vi "Pelletron_Controller.vi"() -> ()   [LabVIEW 2013, in "AccelNET.lvlib" / "Control_VIs.lvlib"]
uses:
  Device IO/Pelletron/Accelnet/Control_VIs.lvlib
  Device IO/Pelletron/Accelnet/Component_Power_Indicator.ctl
  Device IO/Pelletron/Accelnet/Interlocks.ctl
  Device IO/Pelletron/Accelnet/Bypass_Indicator.ctl
  Device IO/Pelletron/Accelnet/Parameters_Indicator.ctl
  Device IO/Pelletron/Accelnet/Parameters_Control.ctl
  Device IO/Pelletron/Accelnet/Conditioning.ctl
  Device IO/Pelletron/Accelnet/Component_Power_Control.ctl
  Device IO/Pelletron/Accelnet/Bypass_Control.ctl
  Controls/PelletronLabview.ctl
  <vilib>/Utility/miscctls.llb/LVPointTypeDef.ctl
  Device IO/Pelletron/Accelnet/TCPinfo.vi
  <userlib>/_OpenG.lib/comparison/comparison.llb/Variant Changed__ogtk.vi
  Device IO/Pelletron/Accelnet/TCP.lvclass
  Device IO/Pelletron/Accelnet/Global_Variables.lvlib
  Device IO/Pelletron/Accelnet/Useful_SubVIs.lvlib
  Device IO/Pelletron/Accelnet/Useful_Controls.lvlib
panel:
  in  "Shut Down":bool
  out "uA/kV":dbl
  in  "Post to database?":bool=TRUE
  out "Connection Status":bool
  out "Bypass Turn Off":dbl format="%<%H:%M:%S>t"
  in  "Synch":bool
  out "Interlock Status":T1
  in  "Y Log Scale?":bool
  in  "X Maximum":dbl max=0.0 step=30.0 format="%<%H:%M:%S>t"
  in  "X Autoscale":bool=TRUE
  in  "X Minimum":dbl max=0.0 step=30.0 format="%<%H:%M:%S>t"
  in  "Y Autoscale":bool=TRUE
  in  "Y Maximum":dbl
  in  "Y Minimum":dbl
  out "Start Time":dbl format="%<%m/%d/%Y  -  %H:%M:%S>T"
  in  "Clear":bool
  out "XY Graph":cluster{dbl[], dbl[]}(graph)
  in  "Plotter Selector":u16(ring) items=["High Voltage", "High Voltage PS", "Chain Current", "Column Current", "Lost Charge", "Radiation", "Pressure", "HV Control Difference"]
  out "Stop Checking for Sparks Start":dbl
  in  "Stop Condition":bool
  in  "Spark Counter Reset":bool
  in  "Update Parameters":bool
  in  "Param Controls":T2 {"Control Reference\nVoltage (MV)" min=0.3 max=3.0 step=0.1; "High Voltage\nPS Setting (kV)" min=0.0 max=18.0 step=0.2; "Spark\nLimit" min=0.0 max=10.0 step=1.0}
  out "Parameters":T3 {"High\nVoltage (MV)" format="%#.4g"; "Control Reference\nVoltage (MV)" format="%#.4g"; "+ High Voltage\nPS (kV)" format="%#.4g"; "- High Voltage\nPS (kV)" format="%#.4g"; "HV Control\nDifference (kV)" format="%#.4g"; "High Voltage\nPS Setting (kV)" format="%#.4g"; "Chain\nCurrent (uA)" format="%#.4g"; "Column\nCurrent (uA)" format="%#.4g"; "Spark\nLimit" format="%#.0g"; "Spark\nCount" format="%#.0g"; "Lost Charge (uA)" scale=-10.0..10.0; "Spark\nThreshold (MV)" format="%#.4g"; "Radiation (mRad/hr)" step=3.978696e-316 scale=0.02..200.0 scale format="%#.4f"; "Vacuum (Torr)" scale=1e-09..0.001 scale format="%#_6e"}
  out "Warning!":bool
  in  "Reset":bool
  out "Rad. Avg.":dbl(slide) scale=0.02..200.0 scale format="%.0e"
  out "Stopped":bool
  out "Spark\nCounter":i64
  in  "Spark Limit":i64=2
  in  "Emergency Stop":bool
  out "Accelnet Write Errors":errorcluster
  in  "Clear Errors":bool
  out "Accelnet Read Errors":errorcluster
  in  "stop":bool
  out "Condition\nStart Time":dbl format="%<%H:%M:%S>T"
  in  "Conditioning":T4
  in  "Bypass Control":T5
  in  "Update Bypass":bool
  out "Pelletron Bypass":T6
  in  "Component Power Control":T7
  in  "Update On/off":bool
  out "Component\nPower":T8
  # "Instructions:\n\n1) Make sure TCP Control is on and the connection is open.  This is true if you can see TCP information on the top where it says IP Address.\n\n2) Turn on the Pelletron Controller\n\n3) Check to see that the Blower and Ion Gauge Filament is on\n\n4) Check all interlocks are lighte and all bypasses are not.\n\n5) Controls are separate from readings.  Pressing the update button in each respective section sends the commands to the Accelnet system.\n\n6) If the Stopped light is on, then the system will lock out all Pelletron controls and shut off the system until the Reset button is pressed.\n\n7) When finished, stop program with Stop button (make sure Pelletron is off)."
  # "Pelletron Startup Sequence:\n1.  Turn on HV Power Supply\n2. Check +High Voltage PS under parameters to be 1 kV if not change it using the High Voltage PS Setting\n3. Turn on Chain PS\n4. Turn on Chain\n5. Condition Pelletron using auto conditioner or manually using High Voltage PS Setting under Parameter Control\n6.  Check Control Reference Voltage under Parameters to be desired voltage and change it if it is not\n7.  Turn on Control Mode\n8.  Open Beamline Gate Valve\n9.  Turn on Rotating Shaft\n10. Operate Pelletron source through Andrew's Box"
  # "Pelletron Shutdown Sequence:\n1.  Make sure Andrew's box is turned down and off\n2.  Turn off Rotating Shaft\n3.  Close Beamline Gatevalve\n         a.  If you are leaving the pelletron on but the accelerator off, stop here.\n4. Check High Voltage PS Setting to be close to + High Voltage PS, if not set it to ~0.2kV above the current setting\n5.  Turn off Control Mode\n6.  Set Voltage to 1 kv using HighVoltage PS Setting\n7.  Reset spark counter after you see the spark count rise by one by hitting the Spark Reset Button.\n8.  Turn off Chain\n9.  Turn off Chain PS and HV Power Supply\n10.  Stop the program."
  # "Interlocks"
  # "Pelletron Plotter"
  # "Parameter Control"
  # "Parameters"
  # "LabVIEW Interlocks"
  # "Pelletron\n   Stop"
  # "Conditioning"
  # "Bypass"
  # "Component On/Off"
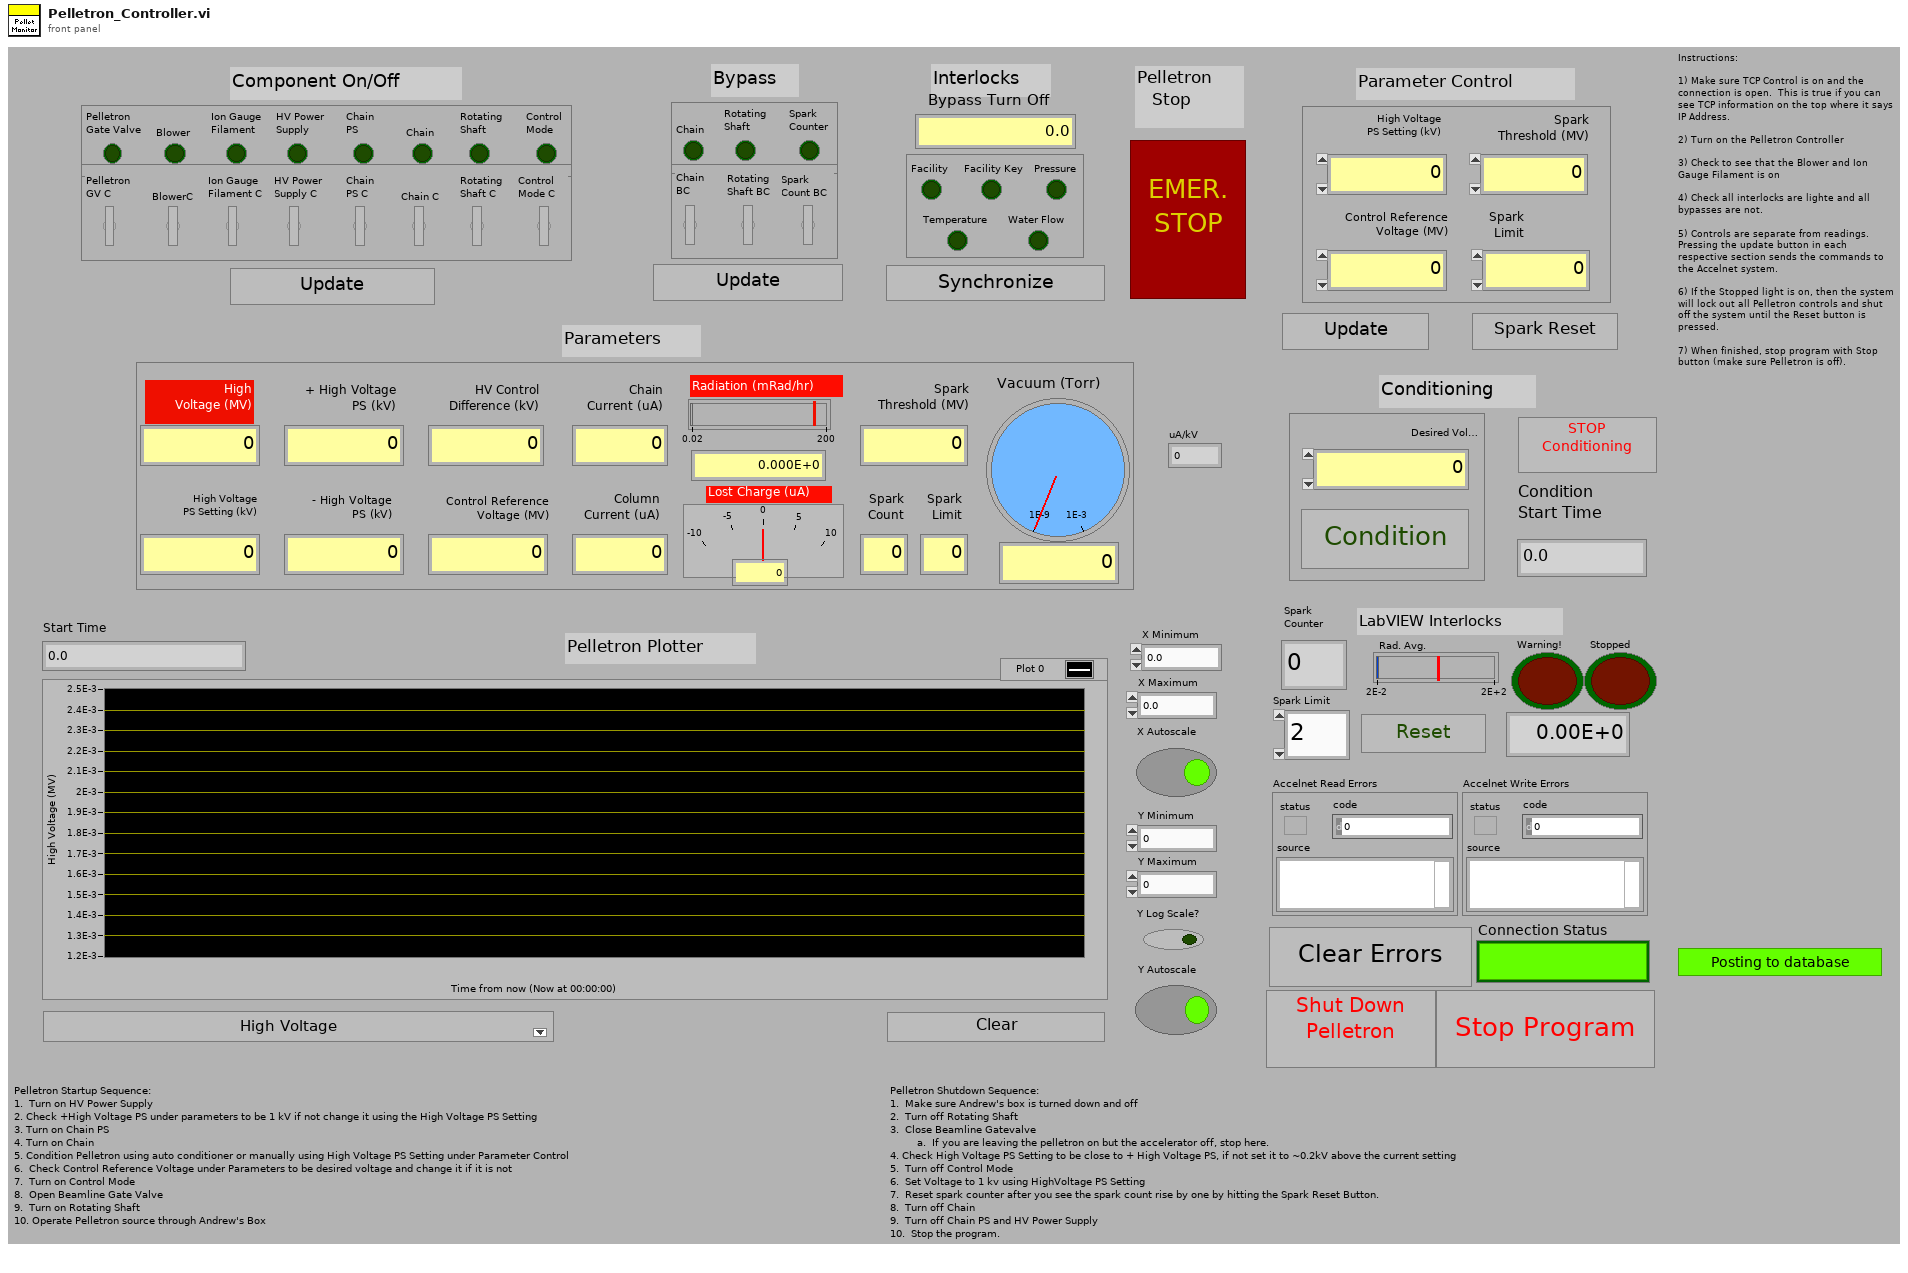
[diagram p1: front panel]
types:
  T1 = typedef "AccelNET.lvlib/Useful_Controls.lvlib/Interlocks.ctl" = cluster{"Facility":bool, "Facility Key":bool, "Water Flow":bool, "Pressure":bool, "Temperature":bool}
  T2 = typedef "AccelNET.lvlib/Useful_Controls.lvlib/Parameters_Control.ctl" = cluster{"Spark\nThreshold (MV)":dbl, "Spark\nLimit":dbl, "High Voltage\nPS Setting (kV)":dbl, "Control Reference\nVoltage (MV)":dbl}
  T3 = typedef "AccelNET.lvlib/Useful_Controls.lvlib/Parameters_Indicator.ctl" = cluster{"Vacuum (Torr)":dbl, "Radiation (mRad/hr)":dbl, "Spark\nThreshold (MV)":dbl, "Lost Charge (uA)":dbl, "Spark\nCount":dbl, "Spark\nLimit":dbl, "Column\nCurrent (uA)":dbl, "Chain\nCurrent (uA)":dbl, "High Voltage\nPS Setting (kV)":dbl, "HV Control\nDifference (kV)":dbl, "- High Voltage\nPS (kV)":dbl, "+ High Voltage\nPS (kV)":dbl, "Control Reference\nVoltage (MV)":dbl, "High\nVoltage (MV)":dbl}
  T4 = typedef "AccelNET.lvlib/Useful_Controls.lvlib/Conditioning.ctl" = cluster{"Desired Voltage (MV)":dbl, "Conditioning?":bool}
  T5 = typedef "AccelNET.lvlib/Useful_Controls.lvlib/Bypass_Control.ctl" = cluster{"Chain\nBC":bool, "Rotating\nShaft BC":bool, "Spark\nCount BC":bool}
  T6 = typedef "AccelNET.lvlib/Useful_Controls.lvlib/Bypass_Indicator.ctl" = cluster{"Chain":bool, "Rotating\nShaft":bool, "Spark\nCounter":bool}
  T7 = typedef "AccelNET.lvlib/Useful_Controls.lvlib/Component_Power_Control.ctl" = cluster{"Pelletron\nGV C":bool, "BlowerC":bool, "Chain C":bool, "Rotating\nShaft C":bool, "HV Power\nSupply C":bool, "Ion Gauge\nFilament C":bool, "Control\nMode C":bool, "Chain\nPS C":bool}
  T8 = typedef "AccelNET.lvlib/Useful_Controls.lvlib/Component_Power_Indicator.ctl" = cluster{"Pelletron\nGate Valve":bool, "Blower":bool, "Chain":bool, "Rotating\nShaft":bool, "HV Power\nSupply":bool, "Ion Gauge\nFilament":bool, "Control\nMode":bool, "Chain\nPS":bool}
  T9 = typedef "LVPointTypeDef.ctl" = cluster{"Horizontal":i16, "Vertical":i16}
  T10 = typedef "PelletronLabview.ctl" = cluster{"Timestamp":timestamp, "High Voltage":sgl, "+ High Voltage Supply":dbl, "- High Voltage Supply":dbl, "HV Control Difference":dbl, "Vacuum Pressure":sgl, "Radiation":dbl, "Column Current":sgl, "Lost Charge":dbl, "Chain Current":sgl, "Control High Voltage":dbl}
  T11 = cluster{"Time":dbl, "High Voltage":dbl, "High VoltagePS":dbl, "Chain Current":dbl, "Column Current":dbl, "Lost Charge":dbl, "Radiation":dbl, "Pressure":dbl, "HV Control Difference":dbl}[]
  T12 = cluster{"Spark\nThreshold (MV)":dbl, "Spark\nLimit":dbl, "High Voltage\nPS Setting (kV)":dbl, "Control Reference\nVoltage (MV)":dbl}
  T13 = enum8{"Enabled", "Disabled", "Disabled and Grayed Out"}
  T14 = cluster{"Time":dbl, "High Voltage":dbl, "High VoltagePS":dbl, "Chain Current":dbl, "Column Current":dbl, "Lost Charge":dbl, "Radiation":dbl, "Pressure":dbl, "HV Control Difference":dbl}
  T15 = cluster{"High\nVoltage (MV)":dbl, "Vacuum (Torr)":dbl, "Lost Charge (uA)":dbl, "+ High Voltage\nPS (kV)":dbl}
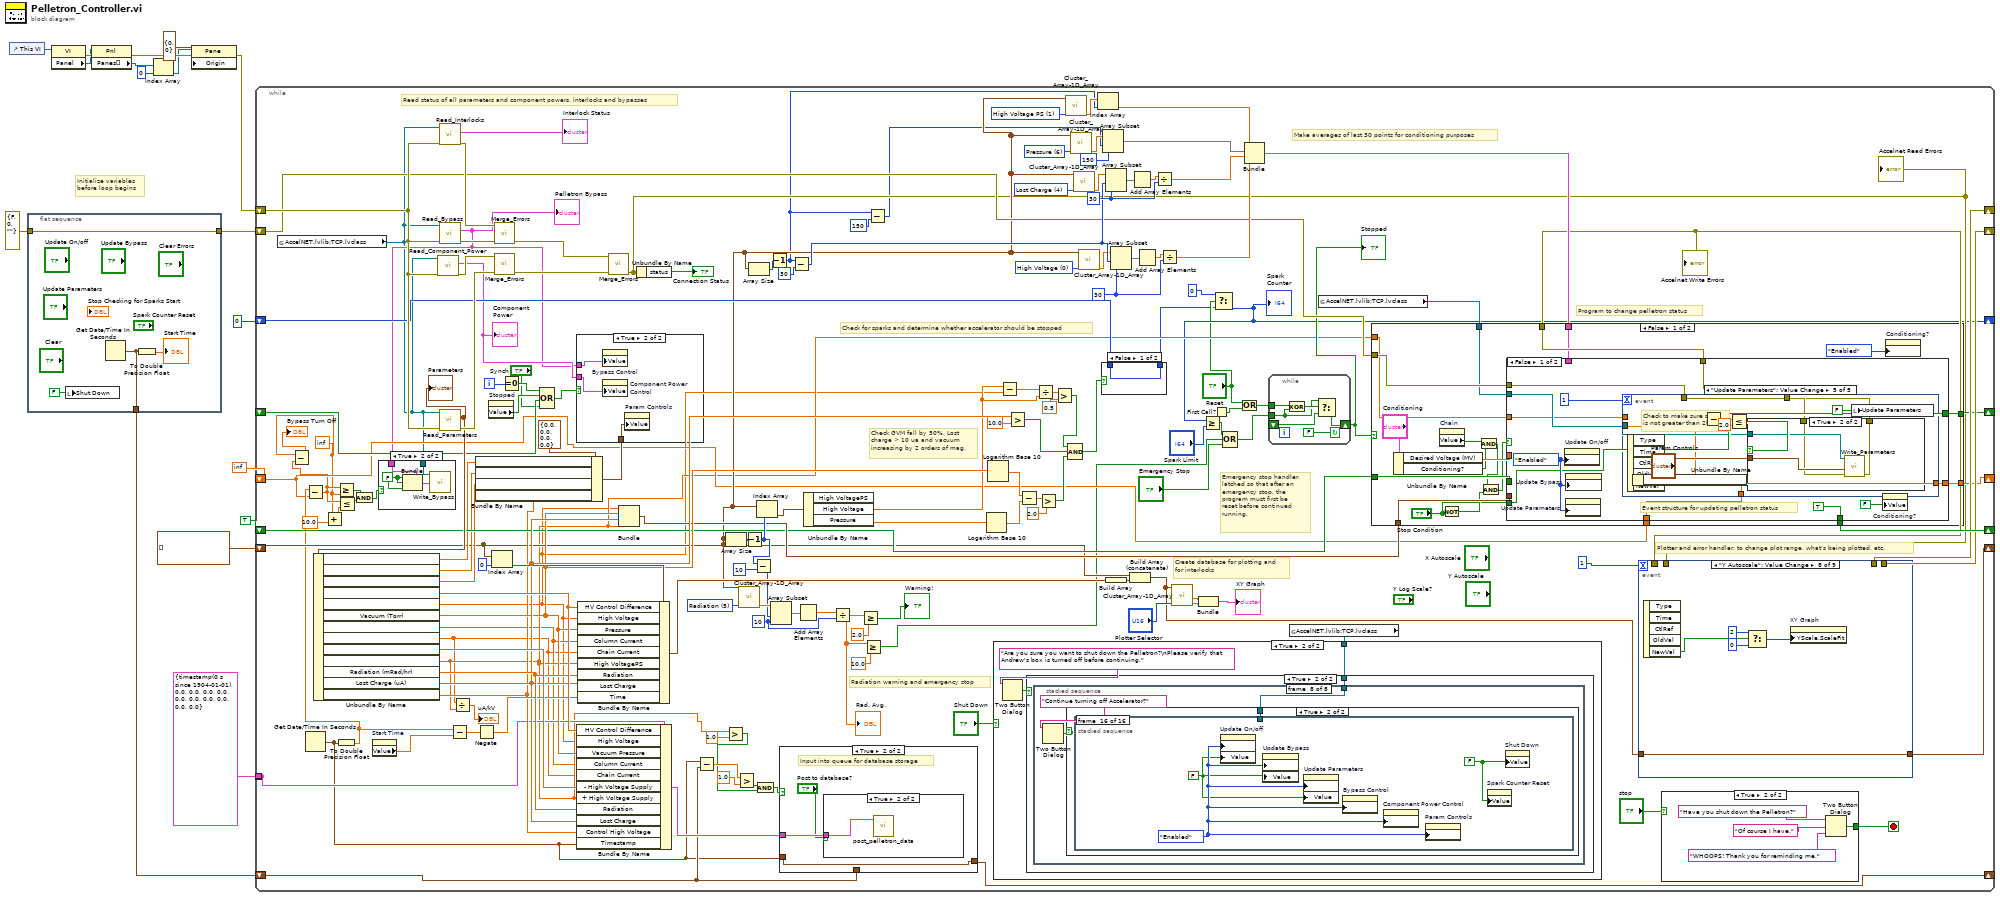
[diagram p0: block diagram]
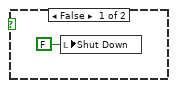
[diagram p3: hidden frame]
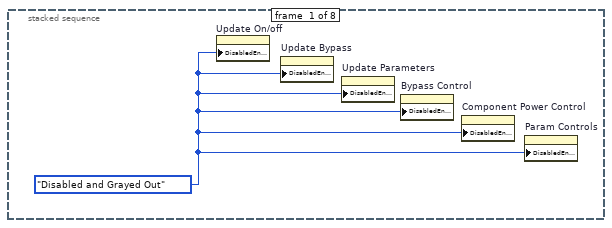
[diagram p4: hidden frame]
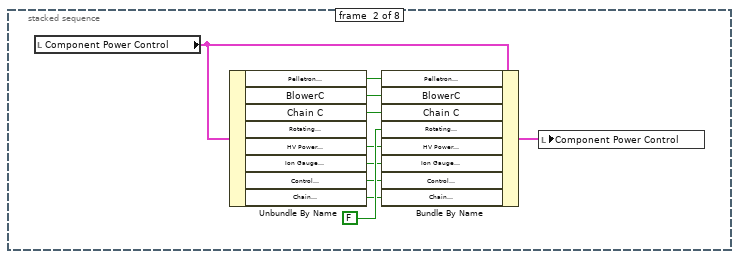
[diagram p5: hidden frame]
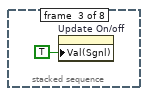
[diagram p6: hidden frame]
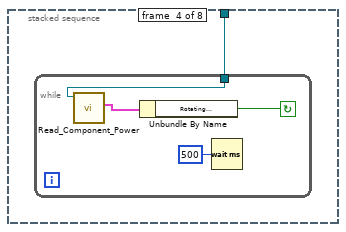
[diagram p7: hidden frame]
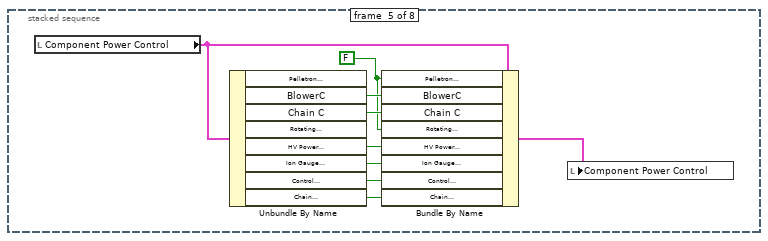
[diagram p8: hidden frame]
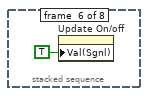
[diagram p9: hidden frame]
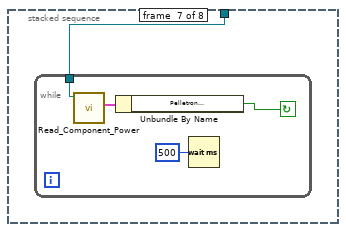
[diagram p10: hidden frame]
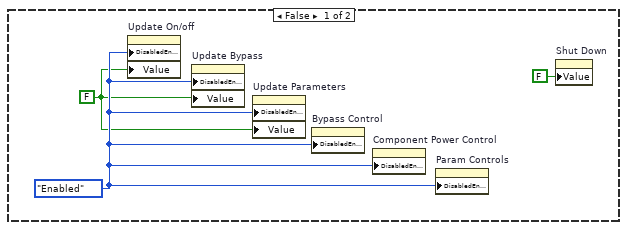
[diagram p11: hidden frame]
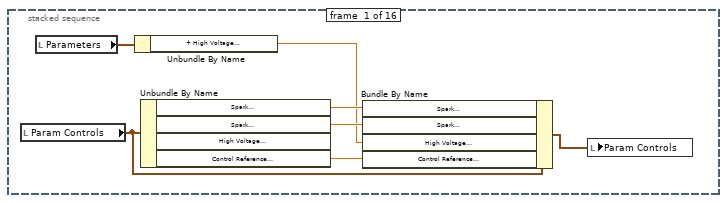
[diagram p12: hidden frame]
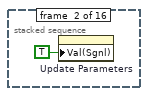
[diagram p13: hidden frame]
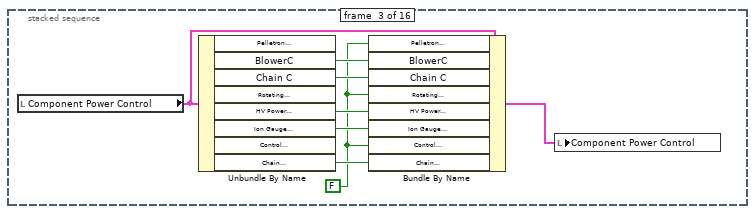
[diagram p14: hidden frame]
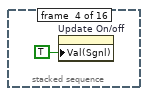
[diagram p15: hidden frame]
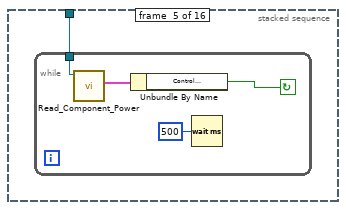
[diagram p16: hidden frame]
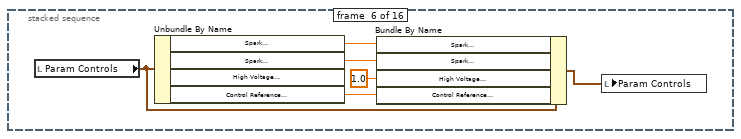
[diagram p17: hidden frame]
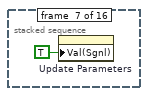
[diagram p18: hidden frame]
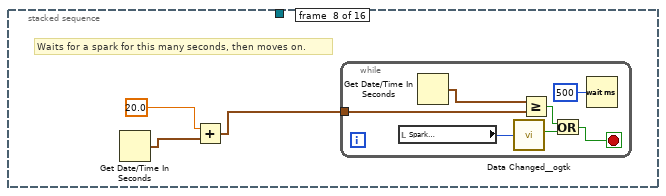
[diagram p19: hidden frame]
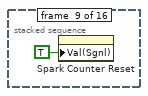
[diagram p20: hidden frame]
diagram:
  # "Initialize variables\nbefore loop begins"
  n1 = control-ref of="This VI"() -> (w12:refnum<vi>)
  n2 = flat-sequence {
    tunnel: [w21] -> w1
    tunnel: [w19] -> w2
    tunnel: errorcluster {"status"=FALSE, "code"=0, "source"=""} ("error out") -> [w21]
    frame #0 {
      n3 = local write "Shut Down"(FALSE ("Shut Down")) -> ()
      n4 = Get Date/Time In Seconds() -> (seconds since 1Jan1904=w19:timestamp)
      n5 = To Double Precision Float(number=w19) -> (double precision float=→"Start Time":dbl)
    }
  }
  n6 = property class="VI"(reference=w12) -> (error out=w11:errorcluster, "Panel"=w10:refnum<vi>)  [unwired: 1 in, 1 out]
  n7 = property class="Pnl"(reference=w10, error in=w11) -> (error out=w9:errorcluster, "Panes[]"=w8:refnum<vi>[])  [unwired: 1 out]
  n8 = Index Array(array=w8, index=0) -> (element=w6:refnum<vi>)
  n9 = property class="Pane"(reference=w6, error in=w9, "Origin"=T9 {"Horizontal"=0, "Vertical"=0}) -> (error out=w4:errorcluster)  [unwired: 1 out]
  n10 = while {
    shift-right: [w108] -> _
    shift-left: w4 -> [w174]
    shift-right: [w159] -> _
    shift-left: T11 [] -> [w92]
    shift-right: [w26] -> _
    shift-left: i64 0 -> [w138]
    shift-right: [w107] -> _
    shift-left: w1 -> [w97]
    shift-right: [w111] -> _
    shift-left: TRUE -> [w112]
    shift-right: [w70] -> _
    shift-left: _ -> [w69]
    shift-right: [w67] -> _
    shift-left: inf -> [w65]
    tunnel: [w48] -> _
    tunnel: T10 {"Timestamp"=timestamp(0 s since 1904-01-01), "High Voltage"=0.0, "+ High Voltage Supply"=0.0, "- High Voltage Supply"=0.0, "HV Control Difference"=0.0, "Vacuum Pressure"=0.0, "Radiation"=0.0, "Column Current"=0.0, "Lost Charge"=0.0, "Chain Current"=0.0, "Control High Voltage"=0.0} ("Cluster") -> [w48]
    shift-right: [w30] -> _
    shift-left: w2 -> [w44]
    i -> [w106]
    stop <- w29 stop-if-true
    w52 = inf ("y")
    w114 = u16 1 items=["High Voltage", "High Voltage PS", "Chain Current", "Column Current", "Lost Charge", "Radiation", "Pressure", "HV Control Difference"] ("Plotter Selector")
    w123 = u16 6 items=["High Voltage", "High Voltage PS", "Chain Current", "Column Current", "Lost Charge", "Radiation", "Pressure", "HV Control Difference"] ("Plotter Selector")
    w124 = 30 ("length")
    w127 = u16 4 items=["High Voltage", "High Voltage PS", "Chain Current", "Column Current", "Lost Charge", "Radiation", "Pressure", "HV Control Difference"] ("Plotter Selector")
    w130 = 30 ("length")
    w135 = u16 0 items=["High Voltage", "High Voltage PS", "Chain Current", "Column Current", "Lost Charge", "Radiation", "Pressure", "HV Control Difference"] ("Plotter Selector")
    w134 = 10 ("length")
    w148 = u16 5 items=["High Voltage", "High Voltage PS", "Chain Current", "Column Current", "Lost Charge", "Radiation", "Pressure", "HV Control Difference"] ("Plotter Selector")
    # "Emergency stop handler,\nlatched so that after an\nemergency stop, the \nprogram must first be \nreset before continued\nrunning."
    # "Plotter and error handler, to change plot range, what's being plotted, etc."
    # "Program to change pelletron status"
    # "Make averages of last 30 points for conditioning purposes"
    # "Check GVM fall by 50%, Lost\ncharge > 10 ua and vacuum\nincreasing by 2 orders of mag."
    # "Create database for plotting and\nfor interlocks"
    # "Radiation warning and emergency stop"
    # "Check for sparks and determine whether accelerator should be stopped"
    # "Read status of all parameters and component powers, interlocks and bypasses"
    n11 = global read "TCPinfo.vi" "AccelNET.lvlib:TCP.lvclass"() -> (w61:refnum<class "TCP.lvclass">)
    n12 = Get Date/Time In Seconds() -> (seconds since 1Jan1904=w43:timestamp)
    n13 = Add(x=w52, y=10.0) -> (x+y=w54:dbl)
    n14 = To Double Precision Float(number=w43) -> (double precision float=w66:dbl)
    n15 = Subtract(x=w66, y=w65) -> (x-y=w59:dbl)
    n16 = Subtract(x=w52, y=w59) -> (x-y=→"Bypass Turn Off":dbl)
    n17 = Greater Or Equal?(x=w59, y=w52) -> (x >= y?=w64:bool)
    n18 = Less Or Equal?(x=w59, y=w54) -> (x <= y?=w63:bool)
    n19 = And(x=w64, y=w63) -> (x .and. y?=w55:bool)
    n20 = property on="Start Time" class="DigNum (strict)"() -> ("Value"=w167:dbl)  [unwired: 2 in, 2 out]
    n21 = call "Read_Component_Power.vi"("error in (no error)"=w174, "AccelNET.lvlib:TCP.lvclass"=w61) -> ("Error Out"=w171:errorcluster, "Component Power"=w68:T8)  [unwired: 8 in]
    "Component\nPower" <- w68
    n22 = call "Read_Interlocks.vi"("Error In"=w174, "AccelNET.lvlib:TCP.lvclass"=w61) -> ("Error Out"=w173:errorcluster, "Interlock Status"=→"Interlock Status":T1)  [unwired: 8 in]
    n23 = call "Read_Bypass.vi"("error in (no error)"=w174, "AccelNET.lvlib:TCP.lvclass"=w61) -> ("Error Out"=w172:errorcluster, "Pelletron Bypass"=w62:T6)  [unwired: 8 in]
    "Pelletron Bypass" <- w62
    n24 = case shown="True" w55 {
      tunnel: w62 -> [_ w301]
      tunnel: w61 -> [_ w298]
      frame False {
      }
      frame True {
        w300 = FALSE ("Chain")
        n25 = Bundle(cluster=w301, "Chain"=w300, "Rotating\nShaft"=w300, "Spark\nCounter"=w300) -> (w299:T6)
        n26 = call "Write_Bypass.vi"("AccelNET.lvlib:TCP.lvclass"=w298, "Pelletron Bypass"=w299) -> ()  [unwired: 8 in, 1 out]
      }
    }
    n27 = call "Read_Parameters.vi"("error in (no error)"=w174, "AccelNET.lvlib:TCP.lvclass"=w61) -> ("Error Out"=w170:errorcluster, "Parameters"=w165:T3)  [unwired: 8 in]
    "Parameters" <- w165
    n28 = Unbundle By Name(w165) -> ("Spark\nThreshold (MV)"=w99:dbl, "Spark\nLimit"=w100:dbl, "High Voltage\nPS Setting (kV)"=w101:dbl, "HV Control\nDifference (kV)"=w153:dbl, "High\nVoltage (MV)"=w34:dbl, "Vacuum (Torr)"=w116:dbl, "Column\nCurrent (uA)"=w36:dbl, "Chain\nCurrent (uA)"=w35:dbl, "- High Voltage\nPS (kV)"=w154:dbl, "+ High Voltage\nPS (kV)"=w38:dbl, "Radiation (mRad/hr)"=w152:dbl, "Lost Charge (uA)"=w117:dbl, "Control Reference\nVoltage (MV)"=w102:dbl)
    n29 = Subtract(x=w66, y=w167) -> (x-y=w156:dbl)
    n30 = Divide(x=w35, y=w38) -> (x/y=→"uA/kV":dbl)
    n31 = Bundle By Name(cluster=T12 {"Spark\nThreshold (MV)"=0.0, "Spark\nLimit"=0.0, "High Voltage\nPS Setting (kV)"=0.0, "Control Reference\nVoltage (MV)"=0.0}, "Spark\nThreshold (MV)"=w99, "Spark\nLimit"=w100, "High Voltage\nPS Setting (kV)"=w101, "Control Reference\nVoltage (MV)"=w102) -> (w103:T12)
    n32 = Negate(x=w156) -> (-x=w151:dbl)
    n33 = property on="Stopped" class="Bool (strict)"() -> ("Value"=w77:bool)  [unwired: 2 in, 2 out]
    n34 = Index Array(array=w92, index=0) -> (element=w157:T14)
    n35 = call "Merge_Errors.vi"("Error 2"=w172, "Error 1"=w173) -> ("Error Out"=w169:errorcluster)  [unwired: 9 in]
    n36 = call "Merge_Errors.vi"("Error 2"=w170, "Error 1"=w171) -> ("Error Out"=w168:errorcluster)  [unwired: 9 in]
    n37 = Equal To 0?(x=w106) -> (x = 0?=w76:bool)
    n38 = Compound Arithmetic op=OR(w76, w77, w69, "Synch") -> (w75:bool)
    n39 = case shown="True" w75 {
      tunnel: w68 -> [_ w309]
      tunnel: w62 -> [_ w310]
      tunnel: w103 -> [_ w308]
      frame False {
      }
      frame True {
        n40 = property on="Bypass Control" class="Clust (strict)"("Value"=w310) -> ()  [unwired: 2 in, 2 out]
        n41 = property on="Component Power Control" class="Clust (strict)"("Value"=w309) -> ()  [unwired: 2 in, 2 out]
        n42 = property on="Param Controls" class="Clust (strict)"("Value"=w308) -> ()  [unwired: 2 in, 2 out]
      }
    }
    n43 = Bundle By Name(cluster=w48, "HV Control Difference"=w153, "High Voltage"=w34, "Vacuum Pressure"=w116, "Column Current"=w36, "Chain Current"=w35, "- High Voltage Supply"=w154, "+ High Voltage Supply"=w38, "Radiation"=w152, "Lost Charge"=w117, "Control High Voltage"=w102, "Timestamp"=w43) -> (w47:T10)
    n44 = Bundle By Name(cluster=w157, "HV Control Difference"=w153, "High Voltage"=w34, "Pressure"=w116, "Column Current"=w36, "Chain Current"=w35, "High VoltagePS"=w38, "Radiation"=w152, "Lost Charge"=w117, "Time"=w151) -> (w160:T14)
    n45 = call "Merge_Errors.vi"("Error 2"=w168, "Error 1"=w169) -> ("Error Out"=w57:errorcluster)  [unwired: 9 in]
    "Accelnet Read Errors" <- w57
    n46 = Bundle("High\nVoltage (MV)"=w34, "Vacuum (Torr)"=w116, "Lost Charge (uA)"=w117, "+ High Voltage\nPS (kV)"=w38) -> (w115:T15)  [unwired: 1 in]
    n47 = Unbundle By Name(w57) -> ("status"=→"Connection Status":bool)
    n48 = Subtract(x=w43, y=w44) -> (x-y=w45:dbl)
    n49 = Greater?(x=w38, y=1.0) -> (0:w40:bool)
    n50 = Array Size(array=w92) -> (size(s)=w150:i32)
    n51 = Greater?(x=w45, y=1.0 ("x")) -> (0:w42:bool)
    n52 = call "Cluster_Array-1D_Array.vi"("Plotter Selector"=w148, "Input Cluster"=w92) -> ("Output Data"=w147:dbl[])  [unwired: 8 in, 1 out]
    n53 = Decrement(x=w150) -> (x-1=w146:i32)
    n54 = Array Size(array=w92) -> (size(s)=w129:i32)
    n55 = Subtract(x=w146, y=10) -> (x-y=w133:i32)
    n56 = And(x=w42, y=w40) -> (x .and. y?=w41:bool)
    n57 = Index Array(array=w92, index=w146) -> (element=w149:T14)
    n58 = Decrement(x=w129) -> (x-1=w50:i32)
    n59 = Array Subset(array=w147, index=w133, length=w134) -> (w144:dbl[])
    n60 = case shown="True" w41 {
      tunnel: w47 -> [_ w296]
      tunnel: w44 -> [w293 _]
      tunnel: [w293 w295] -> w30
      tunnel: w43 -> [_ w295]
      frame False {
      }
      frame True {
        # "Input into queue for database storage"
        n61 = case shown="True" "Post to database?" {
          tunnel: w296 -> [_ w297]
          frame False {
          }
          frame True {
            n62 = call "post_pelletron_data.vi"("Input data"=w297) -> ()  [unwired: 9 in, 1 out]
          }
        }
      }
    }
    n63 = Subtract(x=w50, y=30) -> (x-y=w121:i32)
    n64 = Add Array Elements(numeric array=w144) -> (sum=w143:dbl)
    n65 = Unbundle By Name(w149) -> ("High Voltage"=w79:dbl, "Pressure"=w140:dbl)  [unwired: 1 out]
    n66 = Divide(x=w143, y=w134) -> (x/y=w98:dbl)
    "Rad. Avg." <- w98
    n67 = Greater Or Equal?(x=w98, y=2.0) -> (x >= y?=→"Warning!":bool)
    n68 = Greater Or Equal?(x=w98, y=10.0) -> (x >= y?=w32:bool)
    n69 = Subtract(x=w50, y=150) -> (x-y=w49:i32)
    n70 = Logarithm Base 10(1:w140) -> (0:w86:dbl)
    n71 = Logarithm Base 10(1:w116) -> (0:w87:dbl)
    n72 = Subtract(x=w79, y=w34) -> (x-y=w80:dbl)
    n73 = Greater?(x=w117, y=10.0) -> (0:w82:bool)
    n74 = Subtract(x=w87, y=w86) -> (x-y=w85:dbl)
    n75 = Divide(x=w80, y=w79) -> (x/y=w90:dbl)
    n76 = Greater?(x=w85, y=2.0) -> (0:w83:bool)
    n77 = Greater?(x=w90, y=0.5) -> (0:w81:bool)
    n78 = call "Cluster_Array-1D_Array.vi"("Plotter Selector"=w114, "Input Cluster"=w92) -> ("Output Data"=w71:dbl[])  [unwired: 8 in, 1 out]
    n79 = Compound Arithmetic op=AND(w81, w82, w83) -> (w139:bool)
    n80 = call "Cluster_Array-1D_Array.vi"("Plotter Selector"=w123, "Input Cluster"=w92) -> ("Output Data"=w72:dbl[])  [unwired: 8 in, 1 out]
    n81 = call "Cluster_Array-1D_Array.vi"("Plotter Selector"=w127, "Input Cluster"=w92) -> ("Output Data"=w73:dbl[])  [unwired: 8 in, 1 out]
    n82 = call "Cluster_Array-1D_Array.vi"("Plotter Selector"=w135, "Input Cluster"=w92) -> ("Output Data"=w74:dbl[])  [unwired: 8 in, 1 out]
    n83 = Index Array(array=w71, index=w50) -> (element=w113:dbl)
    n84 = case shown="False" w139 {
      tunnel: w138 -> [w431 w433]
      tunnel: [w431 w432] -> w24
      frame False {
      }
      frame True {
        n85 = Increment(x=w433) -> (x+1=w432:i64)
      }
    }
    n86 = Array Subset(array=w72, index=w49, length=150) -> (w91:dbl[])
    n87 = Array Subset(array=w73, index=w121, length=w124) -> (w126:dbl[])
    n88 = Build Array(w160) -> (w155:T11)
    n89 = Array Subset(array=w74, index=w121, length=w130) -> (w132:dbl[])
    n90 = Build Array (concatenate)(w92, w155) -> (w28:T11)
    n91 = Add Array Elements(numeric array=w126) -> (sum=w125:dbl)
    n92 = Add Array Elements(numeric array=w132) -> (sum=w131:dbl)
    n93 = Divide(x=w125, y=w124) -> (x/y=w120:dbl)
    n94 = Divide(x=w131, y=w130) -> (x/y=w119:dbl)
    n95 = call "Cluster_Array-1D_Array.vi"("Plotter Selector"="Plotter Selector", "Input Cluster"=w28) -> ("Output Data"=w163:dbl[], "Time"=w161:dbl[])  [unwired: 8 in]
    n96 = Bundle("Time"=w161, "Output Data"=w163) -> (→"XY Graph":cluster{"Time":dbl[], "Output Data":dbl[]})  [unwired: 1 in]
    n97 = First Call?() -> (First Call?: T/F=w94:bool)
    n98 = Select(t=i64 0, s="Reset", f=w24) -> (s? t:f=w26:i64)
    "Spark\nCounter" <- w26
    n99 = Greater Or Equal?(x=w26, y="Spark Limit") -> (x >= y?=w110:bool)
    n100 = Compound Arithmetic op=OR(w110, w32, "Emergency Stop") -> (w96:bool)
    n101 = Or(x="Reset", y=w94) -> (x .or. y?=w93:bool)
    n102 = Bundle("Vacuum (Torr)"=w113, w91, w120, w119) -> (w118:cluster{"Vacuum (Torr)":dbl, dbl[], dbl, dbl})  [unwired: 1 in]
    n103 = while {
      shift-right: [w304] -> w95
      shift-left: _ -> [w302]
      tunnel: w96 -> [w305]
      tunnel: w93 -> [w303]
      stop <- FALSE continue-if-true
      n104 = Exclusive Or(1:w305, 2:w303) -> (0:w306:bool)
      n105 = Select(t=w305, s=w306, f=w302) -> (s? t:f=w304:bool)
    }
    "Stopped" <- w95
    n106 = global read "TCPinfo.vi" "AccelNET.lvlib:TCP.lvclass"() -> (w22:refnum<class "TCP.lvclass">)
    n107 = case shown="True" "Shut Down" {
      tunnel: w22 -> [_ w175]
      frame False {
      }
      frame True {
        n108 = Two Button Dialog(message="Are you sure you want to shut down the Pelletron?\nPlease verify that Andrew's box is turned off before continuing.") -> (T button?=w177:bool)  [unwired: 2 in]
        n109 = case shown="True" w177 {
          tunnel: w175 -> [_ w179]
          frame False {
            n110 = local write "Shut Down"(FALSE ("Shut Down")) -> ()
          }
          frame True {
            n111 = stacked-sequence {
              tunnel: w179 -> [_ _ _ w192 _ _ w207 w212]
              frame #0 {
                w180 = T13."Disabled and Grayed Out" ("Disabled")
                n112 = property on="Update On/off" class="Bool (strict)"("DisabledEnum"=w180) -> ()  [unwired: 2 in, 2 out]
                n113 = property on="Update Bypass" class="Bool (strict)"("DisabledEnum"=w180) -> ()  [unwired: 2 in, 2 out]
                n114 = property on="Update Parameters" class="Bool (strict)"("DisabledEnum"=w180) -> ()  [unwired: 2 in, 2 out]
                n115 = property on="Bypass Control" class="Clust (strict)"("DisabledEnum"=w180) -> ()  [unwired: 2 in, 2 out]
                n116 = property on="Component Power Control" class="Clust (strict)"("DisabledEnum"=w180) -> ()  [unwired: 2 in, 2 out]
                n117 = property on="Param Controls" class="Clust (strict)"("DisabledEnum"=w180) -> ()  [unwired: 2 in, 2 out]
              }
              frame #1 {
                n118 = local read "Component Power Control"() -> (w190:T7)
                n119 = Unbundle By Name(w190) -> ("Pelletron\nGV C"=w188:bool, "BlowerC"=w187:bool, "Chain C"=w186:bool, "HV Power\nSupply C"=w185:bool, "Ion Gauge\nFilament C"=w184:bool, "Control\nMode C"=w183:bool, "Chain\nPS C"=w182:bool)  [unwired: 1 out]
                n120 = Bundle By Name(cluster=w190, "Pelletron\nGV C"=w188, "BlowerC"=w187, "Chain C"=w186, "Rotating\nShaft C"=FALSE, "HV Power\nSupply C"=w185, "Ion Gauge\nFilament C"=w184, "Control\nMode C"=w183, "Chain\nPS C"=w182) -> (w181:T7)
                n121 = local write "Component Power Control"(w181) -> ()
              }
              frame #2 {
                n122 = property on="Update On/off" class="Bool (strict)"("Val(Sgnl)"=TRUE ("Value (Signaling)")) -> ()  [unwired: 2 in, 2 out]
              }
              frame #3 {
                n123 = while {
                  tunnel: w192 -> [w195]
                  stop <- w194 continue-if-true
                  n124 = call "Read_Component_Power.vi"("AccelNET.lvlib:TCP.lvclass"=w195) -> ("Component Power"=w196:T8)  [unwired: 9 in, 1 out]
                  n125 = Unbundle By Name(w196) -> ("Rotating\nShaft"=w194:bool)
                  n126 = Wait (ms)(milliseconds to wait=u32 500) -> ()  [unwired: 1 out]
                }
              }
              frame #4 {
                w197 = FALSE
                n127 = local read "Component Power Control"() -> (w205:T7)
                n128 = Unbundle By Name(w205) -> ("BlowerC"=w204:bool, "Chain C"=w203:bool, "HV Power\nSupply C"=w202:bool, "Ion Gauge\nFilament C"=w201:bool, "Control\nMode C"=w200:bool, "Chain\nPS C"=w199:bool)  [unwired: 2 out]
                n129 = Bundle By Name(cluster=w205, "Pelletron\nGV C"=w197, "BlowerC"=w204, "Chain C"=w203, "Rotating\nShaft C"=w197, "HV Power\nSupply C"=w202, "Ion Gauge\nFilament C"=w201, "Control\nMode C"=w200, "Chain\nPS C"=w199) -> (w198:T7)
                n130 = local write "Component Power Control"(w198) -> ()
              }
              frame #5 {
                n131 = property on="Update On/off" class="Bool (strict)"("Val(Sgnl)"=TRUE ("Value (Signaling)")) -> ()  [unwired: 2 in, 2 out]
              }
              frame #6 {
                n132 = while {
                  tunnel: w207 -> [w210]
                  stop <- w209 continue-if-true
                  n133 = call "Read_Component_Power.vi"("AccelNET.lvlib:TCP.lvclass"=w210) -> ("Component Power"=w211:T8)  [unwired: 9 in, 1 out]
                  n134 = Unbundle By Name(w211) -> ("Pelletron\nGate Valve"=w209:bool)
                  n135 = Wait (ms)(milliseconds to wait=u32 500) -> ()  [unwired: 1 out]
                }
              }
              frame #7 {
                n136 = Two Button Dialog(message="Continue turning off Accelerator?") -> (T button?=w213:bool)  [unwired: 2 in]
                n137 = case shown="True" w213 {
                  tunnel: w212 -> [_ w218]
                  frame False {
                    w216 = FALSE ("Shut Down")
                    w217 = T13."Enabled" ("Disabled")
                    n138 = property on="Update On/off" class="Bool (strict)"("DisabledEnum"=w217, "Value"=w216) -> ()  [unwired: 2 in, 2 out]
                    n139 = property on="Update Bypass" class="Bool (strict)"("DisabledEnum"=w217, "Value"=w216) -> ()  [unwired: 2 in, 2 out]
                    n140 = property on="Update Parameters" class="Bool (strict)"("DisabledEnum"=w217, "Value"=w216) -> ()  [unwired: 2 in, 2 out]
                    n141 = property on="Bypass Control" class="Clust (strict)"("DisabledEnum"=w217) -> ()  [unwired: 2 in, 2 out]
                    n142 = property on="Component Power Control" class="Clust (strict)"("DisabledEnum"=w217) -> ()  [unwired: 2 in, 2 out]
                    n143 = property on="Param Controls" class="Clust (strict)"("DisabledEnum"=w217) -> ()  [unwired: 2 in, 2 out]
                    n144 = property on="Shut Down" class="Bool (strict)"("Value"=FALSE ("Shut Down")) -> ()  [unwired: 2 in, 2 out]
                  }
                  frame True {
                    n145 = stacked-sequence {
                      tunnel: w218 -> [_ _ _ _ w236 _ _ _ _ _ _ w267 _ _ w278 _]
                      frame #0 {
                        n146 = local read "Param Controls"() -> (w224:T2)
                        n147 = local read "Parameters"() -> (w225:T3)
                        n148 = Unbundle By Name(w225) -> ("+ High Voltage\nPS (kV)"=w219:dbl)
                        n149 = Unbundle By Name(w224) -> ("Spark\nThreshold (MV)"=w223:dbl, "Spark\nLimit"=w222:dbl, "Control Reference\nVoltage (MV)"=w221:dbl)  [unwired: 1 out]
                        n150 = Bundle By Name(cluster=w224, "Spark\nThreshold (MV)"=w223, "Spark\nLimit"=w222, "High Voltage\nPS Setting (kV)"=w219, "Control Reference\nVoltage (MV)"=w221) -> (w220:T2)
                        n151 = local write "Param Controls"(w220) -> ()
                      }
                      frame #1 {
                        n152 = property on="Update Parameters" class="Bool (strict)"("Val(Sgnl)"=TRUE ("Value (Signaling)")) -> ()  [unwired: 2 in, 2 out]
                      }
                      frame #2 {
                        w227 = FALSE
                        n153 = local read "Component Power Control"() -> (w234:T7)
                        n154 = Unbundle By Name(w234) -> ("BlowerC"=w229:bool, "Chain C"=w230:bool, "HV Power\nSupply C"=w231:bool, "Ion Gauge\nFilament C"=w232:bool, "Chain\nPS C"=w233:bool)  [unwired: 3 out]
                        n155 = Bundle By Name(cluster=w234, "Pelletron\nGV C"=w227, "BlowerC"=w229, "Chain C"=w230, "Rotating\nShaft C"=w227, "HV Power\nSupply C"=w231, "Ion Gauge\nFilament C"=w232, "Control\nMode C"=w227, "Chain\nPS C"=w233) -> (w228:T7)
                        n156 = local write "Component Power Control"(w228) -> ()
                      }
                      frame #3 {
                        n157 = property on="Update On/off" class="Bool (strict)"("Val(Sgnl)"=TRUE ("Value (Signaling)")) -> ()  [unwired: 2 in, 2 out]
                      }
                      frame #4 {
                        n158 = while {
                          tunnel: w236 -> [w239]
                          stop <- w238 continue-if-true
                          n159 = call "Read_Component_Power.vi"("AccelNET.lvlib:TCP.lvclass"=w239) -> ("Component Power"=w240:T8)  [unwired: 9 in, 1 out]
                          n160 = Unbundle By Name(w240) -> ("Control\nMode"=w238:bool)
                          n161 = Wait (ms)(milliseconds to wait=u32 500) -> ()  [unwired: 1 out]
                        }
                      }
                      frame #5 {
                        n162 = local read "Param Controls"() -> (w246:T2)
                        n163 = Unbundle By Name(w246) -> ("Spark\nThreshold (MV)"=w245:dbl, "Spark\nLimit"=w244:dbl, "Control Reference\nVoltage (MV)"=w243:dbl)  [unwired: 1 out]
                        n164 = Bundle By Name(cluster=w246, "Spark\nThreshold (MV)"=w245, "Spark\nLimit"=w244, "High Voltage\nPS Setting (kV)"=1.0 ("High Voltage\nPS Setting (kV)"), "Control Reference\nVoltage (MV)"=w243) -> (w242:T2)
                        n165 = local write "Param Controls"(w242) -> ()
                      }
                      frame #6 {
                        n166 = property on="Update Parameters" class="Bool (strict)"("Val(Sgnl)"=TRUE ("Value (Signaling)")) -> ()  [unwired: 2 in, 2 out]
                      }
                      frame #7 {
                        # "Waits for a spark for this many seconds, then moves on."
                        n167 = Get Date/Time In Seconds() -> (seconds since 1Jan1904=w250:timestamp)
                        n168 = Add(x=20.0, y=w250) -> (x+y=w249:timestamp)
                        n169 = while {
                          tunnel: w249 -> [w253]
                          stop <- w256 stop-if-true
                          n170 = local read "Spark\nCounter"() -> (w257:i64)
                          n171 = Get Date/Time In Seconds() -> (seconds since 1Jan1904=w252:timestamp)
                          n172 = call-poly <userlib>:"Data Changed__ogtk.vi"("Variant"=w257) -> ("Changed"=w255:bool)
                          n173 = Greater Or Equal?(x=w252, y=w253) -> (x >= y?=w254:bool)
                          n174 = Or(x=w254, y=w255) -> (x .or. y?=w256:bool)
                          n175 = Wait (ms)(milliseconds to wait=u32 500) -> ()  [unwired: 1 out]
                        }
                      }
                      frame #8 {
                        n176 = property on="Spark Counter Reset" class="Bool (strict)"("Val(Sgnl)"=TRUE ("Value (Signaling)")) -> ()  [unwired: 2 in, 2 out]
                      }
                      frame #9 {
                        w263 = FALSE ("Chain\nPS C")
                        n177 = local read "Component Power Control"() -> (w264:T7)
                        n178 = Unbundle By Name(w264) -> ("BlowerC"=w259:bool, "HV Power\nSupply C"=w260:bool, "Ion Gauge\nFilament C"=w261:bool, "Chain\nPS C"=w262:bool)  [unwired: 4 out]
                        n179 = Bundle By Name(cluster=w264, "Pelletron\nGV C"=w263, "BlowerC"=w259, "Chain C"=w263, "Rotating\nShaft C"=w263, "HV Power\nSupply C"=w260, "Ion Gauge\nFilament C"=w261, "Control\nMode C"=w263, "Chain\nPS C"=w262) -> (w265:T7)
                        n180 = local write "Component Power Control"(w265) -> ()
                      }
                      frame #10 {
                        n181 = property on="Update On/off" class="Bool (strict)"("Val(Sgnl)"=TRUE ("Value (Signaling)")) -> ()  [unwired: 2 in, 2 out]
                      }
                      frame #11 {
                        n182 = while {
                          tunnel: w267 -> [w270]
                          stop <- w269 continue-if-true
                          n183 = call "Read_Component_Power.vi"("AccelNET.lvlib:TCP.lvclass"=w270) -> ("Component Power"=w271:T8)  [unwired: 9 in, 1 out]
                          n184 = Unbundle By Name(w271) -> ("Chain"=w269:bool)
                          n185 = Wait (ms)(milliseconds to wait=u32 500) -> ()  [unwired: 1 out]
                        }
                      }
                      frame #12 {
                        w272 = FALSE ("Chain\nPS C")
                        n186 = local read "Component Power Control"() -> (w275:T7)
                        n187 = Unbundle By Name(w275) -> ("BlowerC"=w273:bool, "Ion Gauge\nFilament C"=w274:bool)  [unwired: 6 out]
                        n188 = Bundle By Name(cluster=w275, "Pelletron\nGV C"=w272, "BlowerC"=w273, "Chain C"=w272, "Rotating\nShaft C"=w272, "HV Power\nSupply C"=w272, "Ion Gauge\nFilament C"=w274, "Control\nMode C"=w272, "Chain\nPS C"=w272) -> (w276:T7)
                        n189 = local write "Component Power Control"(w276) -> ()
                      }
                      frame #13 {
                        n190 = property on="Update On/off" class="Bool (strict)"("Val(Sgnl)"=TRUE ("Value (Signaling)")) -> ()  [unwired: 2 in, 2 out]
                      }
                      frame #14 {
                        n191 = while {
                          tunnel: w278 -> [w283]
                          stop <- w280 continue-if-true
                          n192 = call "Read_Component_Power.vi"("AccelNET.lvlib:TCP.lvclass"=w283) -> ("Component Power"=w284:T8)  [unwired: 9 in, 1 out]
                          n193 = Unbundle By Name(w284) -> ("Chain\nPS"=w282:bool, "HV Power\nSupply"=w281:bool)
                          n194 = Or(x=w282, y=w281) -> (x .or. y?=w280:bool)
                          n195 = Wait (ms)(milliseconds to wait=u32 500) -> ()  [unwired: 1 out]
                        }
                      }
                      frame #15 {
                        w286 = FALSE ("Shut Down")
                        w285 = FALSE ("Shut Down")
                        w287 = T13."Enabled" ("Disabled")
                        n196 = property on="Update On/off" class="Bool (strict)"("DisabledEnum"=w287, "Value"=w286) -> ()  [unwired: 2 in, 2 out]
                        n197 = property on="Update Bypass" class="Bool (strict)"("DisabledEnum"=w287, "Value"=w286) -> ()  [unwired: 2 in, 2 out]
                        n198 = property on="Update Parameters" class="Bool (strict)"("DisabledEnum"=w287, "Value"=w286) -> ()  [unwired: 2 in, 2 out]
                        n199 = property on="Bypass Control" class="Clust (strict)"("DisabledEnum"=w287) -> ()  [unwired: 2 in, 2 out]
                        n200 = property on="Component Power Control" class="Clust (strict)"("DisabledEnum"=w287) -> ()  [unwired: 2 in, 2 out]
                        n201 = property on="Param Controls" class="Clust (strict)"("DisabledEnum"=w287) -> ()  [unwired: 2 in, 2 out]
                        n202 = property on="Spark Counter Reset" class="Bool (strict)"("Value"=w285) -> ()  [unwired: 2 in, 2 out]
                        n203 = property on="Shut Down" class="Bool (strict)"("Value"=w285) -> ()  [unwired: 2 in, 2 out]
                      }
                    }
                  }
                }
              }
            }
          }
        }
      }
    }
    n204 = global read "TCPinfo.vi" "AccelNET.lvlib:TCP.lvclass"() -> (w136:refnum<class "TCP.lvclass">)
    n205 = case shown="False" w95 {
      tunnel: w97 -> [w328 w407]
      tunnel: [w327 w404] -> w78
      tunnel: w136 -> [w326 w409]
      tunnel: w118 -> [w325 _]
      tunnel: w115 -> [w324 _]
      tunnel: w112 -> [w323 _]
      tunnel: [w322 TRUE] -> w111
      tunnel: w38 -> [w321 _]
      tunnel: [w315 FALSE ("Value")] -> w70
      tunnel: [w312 w400] -> w67
      tunnel: w65 -> [w311 w400]
      frame False {
        n206 = Unbundle By Name("Conditioning") -> ("Desired Voltage (MV)"=w329:dbl, "Conditioning?"=w320:bool)
        n207 = property on="Chain" class="Bool (strict)"() -> ("Value"=w319:bool)  [unwired: 2 in, 2 out]
        n208 = Not(x="Stop Condition") -> (.not. x?=w317:bool)
        n209 = And(x=w319, y=w320) -> (x .and. y?=w318:bool)
        n210 = And(x=w318, y=w317) -> (x .and. y?=w314:bool)
        n211 = case shown="False" w314 {
          tunnel: w329 -> [_ w390]
          tunnel: w328 -> [w338 w392]
          tunnel: [w337 w391] -> w327
          tunnel: w326 -> [w339 w395]
          tunnel: w325 -> [_ w393]
          tunnel: w324 -> [_ w394]
          tunnel: w323 -> [_ w396]
          tunnel: [TRUE w388] -> w322
          tunnel: w321 -> [w336 _]
          tunnel: [w331 w385] -> w315
          tunnel: "Stop Condition" -> [w331 _]
          tunnel: [w333 w386] -> w312
          tunnel: w311 -> [w332 w386]
          frame False {
            w334 = T13."Enabled" ("Disabled")
            # "Event structure for updating pelletron status"
            n212 = property on="Update On/off" class="Bool (strict)"("DisabledEnum"=w334) -> ()  [unwired: 2 in, 2 out]
            n213 = property on="Update Parameters" class="Bool (strict)"("DisabledEnum"=w334) -> ()  [unwired: 2 in, 2 out]
            n214 = property on="Update Bypass" class="Bool (strict)"("DisabledEnum"=w334) -> ()  [unwired: 2 in, 2 out]
            n215 = event shown="[4] \"Update Parameters\": Value Change" {
              selector: _ -> [_ _ _ _ _]
              dyn-events: _ -> [_ _ _ _ _]
              timeout: 1 -> [_ _ _ _ _]
              tunnel: w339 -> [_ w350 w355 w364 w375]
              tunnel: w338 -> [w343 w348 w354 w363 w374]
              tunnel: [w343 w346 w353 w362 w373] -> w337
              tunnel: w336 -> [_ _ _ _ w371]
              tunnel: [w342 w344 w351 w359 w365] -> w333
              tunnel: w332 -> [w342 w344 w351 _ w365]
              event Timeout {
                n216 = event-data() -> ()  [unwired: 1 in, 2 out]
              }
              event "Spark Counter Reset": Value Change {
                w349 = u16 14 items=["GV", "Blower", "Main Power Supply", "Chain Power Supply", "Chain", "Rotating Shaft", "Power Supply Voltage", "Control Mode", "Control Mode Reference", "Chain Bypass", "Rotating Shaft Bypass", "Spark Counter", "Spark Limit", "Threshold", "Spark Counter Reset", "Ion Filament"] ("Write Selector")
                n217 = event-data() -> ()  [unwired: 1 in, 5 out]
                n218 = call "Change_Pelletron_Status.vi"("error in (no error)"=w348, "Write Value"=1.0, "Write Selector"=w349, "AccelNET.lvlib:TCP.lvclass"=w350) -> ("error out"=w346:errorcluster)  [unwired: 7 in]
                n219 = local write "Spark Counter Reset"(FALSE ("Spark Counter Reset")) -> ()
              }
              event "Update On/off": Value Change {
                n220 = event-data() -> ()  [unwired: 1 in, 5 out]
                n221 = call "Write_Component_Power.vi"("AccelNET.lvlib:TCP.lvclass"=w355, "Component Power"="Component Power Control", "error in (no error)"=w354) -> ("Error Out"=w353:errorcluster)  [unwired: 7 in]
                n222 = property on="Update On/off" class="Bool (strict)"("Value"=FALSE ("Update On/off")) -> ()  [unwired: 2 in, 2 out]
              }
              event "Update Bypass": Value Change {
                n223 = event-data() -> ()  [unwired: 1 in, 5 out]
                n224 = call "Write_Bypass.vi"("AccelNET.lvlib:TCP.lvclass"=w364, "Pelletron Bypass"="Bypass Control", "error in (no error)"=w363) -> ("Error Out"=w362:errorcluster)  [unwired: 7 in]
                n225 = Get Date/Time In Seconds() -> (seconds since 1Jan1904=w357:timestamp)
                n226 = To Double Precision Float(number=w357) -> (double precision float=w359:dbl)
                n227 = local write "Update On/off"(FALSE ("Update On/off")) -> ()
                n228 = property on="Update Bypass" class="Bool (strict)"("Value"=FALSE ("Update Bypass")) -> ()  [unwired: 2 in, 2 out]
              }
              event "Update Parameters": Value Change {
                # "Check to make sure step\nis not greater than 2kV"
                n229 = event-data() -> ()  [unwired: 1 in, 5 out]
                n230 = Unbundle By Name("Param Controls") -> ("High Voltage\nPS Setting (kV)"=w370:dbl)
                n231 = Subtract(x=w370, y=w371) -> (x-y=w369:dbl)
                n232 = Less Or Equal?(x=w369, y=2.0) -> (x <= y?=w367:bool)
                n233 = case shown="True" w367 {
                  tunnel: "Param Controls" -> [_ w384]
                  tunnel: w375 -> [_ w383]
                  tunnel: w374 -> [w380 w382]
                  tunnel: [w376 w381] -> w373
                  frame False {
                    n234 = Bundle By Name(cluster=w380, "status"=FALSE, "code"=5001, "source"="Cannot change HV PS by more\nthan 2kV at a time.") -> (w376:errorcluster)
                  }
                  frame True {
                    n235 = call "Write_Parameters.vi"("error in (no error)"=w382, "Param Controls"=w384, "AccelNET.lvlib:TCP.lvclass"=w383) -> ("Error Out"=w381:errorcluster)  [unwired: 8 in]
                  }
                }
                n236 = local write "Update Parameters"(FALSE ("Update Parameters")) -> ()
              }
            }
            n237 = property on="Conditioning?" class="Bool (strict)"("Value"=FALSE) -> ()  [unwired: 2 in, 2 out]
          }
          frame True {
            w387 = T13."Disabled and Grayed Out" ("Disabled")
            # "Store time of last voltage step"
            # "Conditioning program"
            n238 = case shown="True" w396 {
              tunnel: [w397 w398] -> w389
              frame False {
                n239 = property on="Condition\nStart Time" class="DigNum (strict)"() -> ("Value"=w397:dbl)  [unwired: 2 in, 2 out]
              }
              frame True {
                n240 = Get Date/Time In Seconds() -> (seconds since 1Jan1904=w399:timestamp)
                n241 = To Double Precision Float(number=w399) -> (double precision float=w398:dbl)
                "Condition\nStart Time" <- w398
              }
            }
            n242 = call "Pelletron_Conditioning.vi"("Desired Voltage (MV)"=w390, "Condition Start time"=w389, "error in (no error)"=w392, "Input Old Cluster"=w393, "Input New Cluster"=w394, "AccelNET.lvlib:TCP.lvclass"=w395) -> ("Error Out"=w391:errorcluster, "Conditioning?"=w385:bool, "Step Up Voltage?"=w388:bool)  [unwired: 3 in]
            n243 = property on="Conditioning?" class="Bool (strict)"("Value"=w385) -> ()  [unwired: 2 in, 2 out]
            n244 = property on="Update Parameters" class="Bool (strict)"("DisabledEnum"=w387) -> ()  [unwired: 2 in, 2 out]
            n245 = property on="Update Bypass" class="Bool (strict)"("DisabledEnum"=w387) -> ()  [unwired: 2 in, 2 out]
            n246 = property on="Update On/off" class="Bool (strict)"("DisabledEnum"=w387) -> ()  [unwired: 2 in, 2 out]
          }
        }
        n247 = property on="Conditioning?" class="Bool (strict)"("DisabledEnum"=T13."Enabled" ("Disabled")) -> ()  [unwired: 2 in, 2 out]
      }
      frame True {
        w403 = FALSE ("Update Parameters")
        w402 = T13."Disabled and Grayed Out" ("Disabled")
        w410 = u16 0 items=["GV", "Blower", "Main Power Supply", "Chain Power Supply", "Chain", "Rotating Shaft", "Power Supply Voltage", "Control Mode", "Control Mode Reference", "Chain Bypass", "Rotating Shaft Bypass", "Spark Counter", "Spark Limit", "Threshold", "Spark Counter Reset", "Ion Filament"] ("Write Selector")
        w411 = FALSE ("Value")
        w420 = u16 7 items=["GV", "Blower", "Main Power Supply", "Chain Power Supply", "Chain", "Rotating Shaft", "Power Supply Voltage", "Control Mode", "Control Mode Reference", "Chain Bypass", "Rotating Shaft Bypass", "Spark Counter", "Spark Limit", "Threshold", "Spark Counter Reset", "Ion Filament"] ("Write Selector")
        w421 = u16 6 items=["GV", "Blower", "Main Power Supply", "Chain Power Supply", "Chain", "Rotating Shaft", "Power Supply Voltage", "Control Mode", "Control Mode Reference", "Chain Bypass", "Rotating Shaft Bypass", "Spark Counter", "Spark Limit", "Threshold", "Spark Counter Reset", "Ion Filament"] ("Write Selector")
        w423 = u16 2 items=["GV", "Blower", "Main Power Supply", "Chain Power Supply", "Chain", "Rotating Shaft", "Power Supply Voltage", "Control Mode", "Control Mode Reference", "Chain Bypass", "Rotating Shaft Bypass", "Spark Counter", "Spark Limit", "Threshold", "Spark Counter Reset", "Ion Filament"] ("Write Selector")
        w427 = u16 3 items=["GV", "Blower", "Main Power Supply", "Chain Power Supply", "Chain", "Rotating Shaft", "Power Supply Voltage", "Control Mode", "Control Mode Reference", "Chain Bypass", "Rotating Shaft Bypass", "Spark Counter", "Spark Limit", "Threshold", "Spark Counter Reset", "Ion Filament"] ("Write Selector")
        w430 = u16 4 items=["GV", "Blower", "Main Power Supply", "Chain Power Supply", "Chain", "Rotating Shaft", "Power Supply Voltage", "Control Mode", "Control Mode Reference", "Chain Bypass", "Rotating Shaft Bypass", "Spark Counter", "Spark Limit", "Threshold", "Spark Counter Reset", "Ion Filament"] ("Write Selector")
        # "Emergency stop, turns off chain, cps, tps, and control mode and reduces cps to 0 kV, also turns off conditioning status"
        n248 = call "Change_Pelletron_Status.vi"("error in (no error)"=w407, "Write Value"=0.0, "Write Selector"=w430, "AccelNET.lvlib:TCP.lvclass"=w409) -> ("error out"=w426:errorcluster)  [unwired: 7 in]
        n249 = call "Change_Pelletron_Status.vi"("error in (no error)"=w407, "Write Value"=0.0, "Write Selector"=w421, "AccelNET.lvlib:TCP.lvclass"=w409) -> ("error out"=w417:errorcluster)  [unwired: 7 in]
        n250 = call "Change_Pelletron_Status.vi"("error in (no error)"=w407, "Write Value"=1.0, "Write Selector"=w427, "AccelNET.lvlib:TCP.lvclass"=w409) -> ("error out"=w425:errorcluster)  [unwired: 7 in]
        n251 = call "Change_Pelletron_Status.vi"("error in (no error)"=w407, "Write Value"=0.0, "Write Selector"=w423, "AccelNET.lvlib:TCP.lvclass"=w409) -> ("error out"=w418:errorcluster)  [unwired: 7 in]
        n252 = call "Merge_Errors.vi"("Error 2"=w425, "Error 1"=w426) -> ("Error Out"=w415:errorcluster)  [unwired: 9 in]
        n253 = call "Merge_Errors.vi"("Error 2"=w417, "Error 1"=w418) -> ("Error Out"=w414:errorcluster)  [unwired: 9 in]
        n254 = call "Change_Pelletron_Status.vi"("error in (no error)"=w407, "Write Value"=0.0, "Write Selector"=w410, "AccelNET.lvlib:TCP.lvclass"=w409) -> ("error out"=w405:errorcluster)  [unwired: 7 in]
        n255 = call "Change_Pelletron_Status.vi"("error in (no error)"=w407, "Write Value"=0.0, "Write Selector"=w420, "AccelNET.lvlib:TCP.lvclass"=w409) -> ("error out"=w416:errorcluster)  [unwired: 7 in]
        n256 = call "Merge_Errors.vi"("Error 2"=w415, "Error 1"=w416) -> ("Error Out"=w413:errorcluster)  [unwired: 9 in]
        n257 = call "Merge_Errors.vi"("Error 2"=w414, "Error 1"=w413) -> ("Error Out"=w406:errorcluster)  [unwired: 9 in]
        n258 = call "Merge_Errors.vi"("Error 2"=w405, "Error 1"=w406) -> ("Error Out"=w404:errorcluster)  [unwired: 9 in]
        n259 = property on="Conditioning?" class="Bool (strict)"("DisabledEnum"=w402, "Value"=w403) -> ()  [unwired: 2 in, 2 out]
        n260 = property on="Update Parameters" class="Bool (strict)"("DisabledEnum"=w402, "Value"=w403) -> ()  [unwired: 2 in, 2 out]
        n261 = local write "Emergency Stop"(w411) -> ()
        n262 = property on="Spark Counter Reset" class="Bool (strict)"("DisabledEnum"=w402, "Value"=w403) -> ()  [unwired: 2 in, 2 out]
        n263 = property on="Update Bypass" class="Bool (strict)"("DisabledEnum"=w402, "Value"=w403) -> ()  [unwired: 2 in, 2 out]
        n264 = property on="Update On/off" class="Bool (strict)"("DisabledEnum"=w402, "Value"=w403) -> ()  [unwired: 2 in, 2 out]
        n265 = property on="Conditioning?" class="Bool (strict)"("Value"=w411) -> ()  [unwired: 2 in, 2 out]
      }
    }
    "Accelnet Write Errors" <- w78
    n266 = event shown="[7] \"Y Autoscale\": Value Change" {
      selector: _ -> [_ _ _ _ _ _ _ _ _]
      dyn-events: _ -> [_ _ _ _ _ _ _ _ _]
      timeout: 1 -> [_ _ _ _ _ _ _ _ _]
      tunnel: w28 -> [w436 w440 w441 _ w455 w458 w471 w472 w482]
      tunnel: [w436 w440 w441 T11 [] w455 w458 w471 w472 w482] -> w159
      tunnel: w78 -> [w434 _ _ w446 w453 w462 w469 _ w479]
      tunnel: w57 -> [w435 _ _ w447 w454 w463 w470 _ w480]
      tunnel: [w435 errorcluster {"status"=FALSE, "code"=0, "source"=""} ("Error Out") _ w447 w454 w463 w470 _ w480] -> w108
      tunnel: [w434 errorcluster {"status"=FALSE, "code"=0, "source"=""} ("Error Out") _ w446 w453 w462 w469 _ w479] -> w107
      event Timeout {
        n267 = event-data() -> ()  [unwired: 1 in, 2 out]
      }
      event "Clear Errors": Value Change {
        n268 = event-data() -> ()  [unwired: 1 in, 5 out]
        n269 = invoke on="Accelnet Write Errors" class="Clust (strict)" method="Reinit To Default"() -> ()  [unwired: 3 in, 3 out]
        n270 = invoke on="Accelnet Read Errors" class="Clust (strict)" method="Reinit To Default"() -> ()  [unwired: 3 in, 3 out]
        n271 = local write "Clear Errors"(FALSE ("Clear Errors")) -> ()
      }
      event "Y Log Scale?": Value Change {
        n272 = event-data() -> ("NewVal"=w443:bool)  [unwired: 1 in, 4 out]
        n273 = Select(t=u8 1, s=w443, f=u8 0) -> (s? t:f=w444:u8)
        n274 = property on="XY Graph" class="XYGraph (strict)"("YScale.Mapping Mode"=w444) -> ()  [unwired: 2 in, 2 out]
      }
      event "Clear": Value Change {
        n275 = event-data() -> ()  [unwired: 1 in, 5 out]
        n276 = Get Date/Time In Seconds() -> (seconds since 1Jan1904=w450:timestamp)
        n277 = To Double Precision Float(number=w450) -> (double precision float=w449:dbl)
        n278 = local write "Start Time"(w449) -> ()
      }
      event "X Maximum", "X Minimum": Value Change {
        n279 = event-data() -> ()  [unwired: 1 in, 5 out]
        n280 = property on="XY Graph" class="XYGraph (strict)"("XScale.Maximum"="X Maximum", "XScale.Minimum"="X Minimum", "XScale.ScaleFit"=u8 0 ("X Scale.Scale Fit")) -> ()  [unwired: 2 in, 2 out]
        n281 = local write "X Autoscale"(FALSE ("X Autoscale")) -> ()
      }
      event "Y Maximum", "Y Minimum": Value Change {
        n282 = event-data() -> ()  [unwired: 1 in, 5 out]
        n283 = property on="XY Graph" class="XYGraph (strict)"("YScale.Maximum"="Y Maximum", "YScale.Minimum"="Y Minimum", "YScale.ScaleFit"=u8 0 ("Y Scale.Scale Fit")) -> ()  [unwired: 2 in, 2 out]
        n284 = local write "Y Autoscale"(FALSE ("Y Autoscale")) -> ()
      }
      event "X Autoscale": Value Change {
        n285 = event-data() -> ("NewVal"=w466:bool)  [unwired: 1 in, 4 out]
        n286 = Select(t=2, s=w466, f=0) -> (s? t:f=w465:i32)
        n287 = property on="XY Graph" class="XYGraph (strict)"("XScale.ScaleFit"=w465) -> ()  [unwired: 2 in, 2 out]
      }
      event "Y Autoscale": Value Change {
        n288 = event-data() -> ("NewVal"=w476:bool)  [unwired: 1 in, 4 out]
        n289 = Select(t=u8 2, s=w476, f=u8 0) -> (s? t:f=w473:u8)
        n290 = property on="XY Graph" class="XYGraph (strict)"("YScale.ScaleFit"=w473) -> ()  [unwired: 2 in, 2 out]
      }
      event "Plotter Selector": Value Change {
        n291 = event-data() -> ("NewVal"=w483:u16)  [unwired: 1 in, 4 out]
        n292 = case shown="7" w483 {
          tunnel: [0 0 0 0 0 1 1 0] -> w478
          tunnel: ["High Voltage (MV)" "High Voltage Power Supply (kV)" "Chain Current (uA)" "Column Current (uA)" "Lost Charge (uA)" "Radiation (mRad/hr)" "Pressure (torr)" "HV Control Difference (kV)"] -> w481
          frame 0, Default {
          }
          frame 1 {
          }
          frame 2 {
          }
          frame 3 {
          }
          frame 4 {
          }
          frame 5 {
          }
          frame 6 {
          }
          frame 7 {
          }
        }
        n293 = Not Equal To 0?(x=w478) -> (x != 0?=w477:bool)
        n294 = property on="XY Graph" class="XYGraph (strict)"("YScale.Mapping Mode"=w478, "YScale.NameLbl.Text"=w481) -> ()  [unwired: 2 in, 2 out]
        n295 = local write "Y Log Scale?"(w477) -> ()
      }
    }
    n296 = case shown="True" "stop" {
      tunnel: [FALSE ("T button?") w292] -> w29
      frame False {
      }
      frame True {
        n297 = Two Button Dialog(message="Have you shut down the Pelletron?", 1:"WHOOPS! Thank you for reminding me." ("T button name (\"OK\")"), 2:"Of course I have." ("T button name (\"OK\")")) -> (T button?=w292:bool)
      }
    }
  }
